vi "ReadWrite.Data.vi"(8 "error in":errorcluster, 10 "timeout ms":i32, 11 "Ref":T1) -> (0 "error out":errorcluster, 1 "Timeout?":bool, 2 "Data":dbl[](array[numeric]), 3 "Detect?":bool[](array[boolean]))   [LabVIEW 2026, in "Data Access Engine (Express).lvlib" / "Data Access Engine (Express).lvclass"]
uses:
  Data Access Engine (Express).lvclass
  Access Type Classes/ReadWrite/ReadWrite.lvclass
  Access Type Classes/ReadWrite/ReadWrite.lvclass/ReadWrite.ctl
  Types/ReadWrite.DVR.ctl
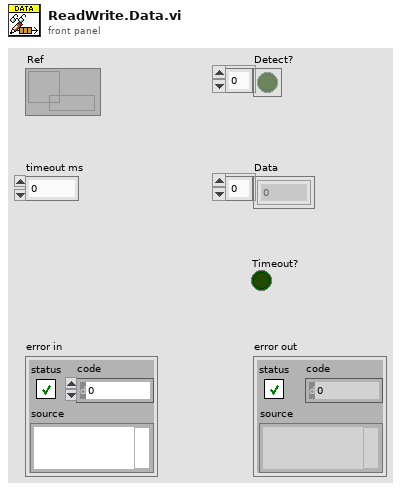
[diagram p1: front panel]
types:
  T1 = typedef "Data Access Engine (Express).lvlib/Data Access Engine (Express).lvclass/ReadWrite.DVR.ctl" = refnum<data-value>
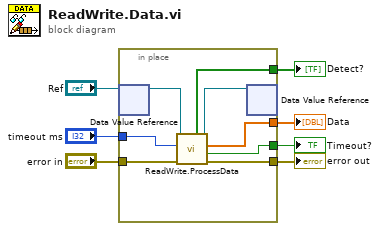
[diagram p0: block diagram]
diagram:
  n1 = in-place {
    in-place-border: "error in" -> [w13]
    in-place-border: [w12] -> w6
    in-place-border: "timeout ms" -> [w11]
    in-place-border: [w10] -> w3
    in-place-border: [w9] -> w2
    in-place-border: [w8] -> w1
    n2 = in-place-dvr #1("Ref") -> (w15:refnum<class "ReadWrite.lvclass">)  [unwired: 1 out]
    n3 = call "ReadWrite.ProcessData.vi"("error in (no error)"=w13, "timeout ms"=w11, "ReadWrite in"=w15) -> ("error out"=w12:errorcluster, "Timeout?"=w9:bool, "Values"=w10:dbl[], "ReadWrite out"=w14:refnum<class "ReadWrite.lvclass">, "Detect?"=w8:bool[])  [unwired: 4 in]
    n4 = in-place-dvr #1(w14) -> ()  [unwired: 2 out]
  }
  "error out" <- w6
  "Data" <- w3
  "Timeout?" <- w2
  "Detect?" <- w1
